vi "Tracer_ClassAttributes.vi"() -> ()   [LabVIEW 2018, in "TracerLibrary.lvlib" / "Tracer.lvclass"]
uses:
  Tracer.lvclass
  Tracer_ObjectAttributes.ctl
panel:
  in  "Max Input Size":i32=200
  in  "Enable Global Tracing":bool
  in  "UpdateCount":i32
  in  "Max Interal Trace Size":i32=-1
  in  "TraceQueues":refnum<queue>[](array[refnum])
  in  "Class Attributes":refnum<data-value>
  # "Trace items"
  # "VI start control trace"
  # "Queue data"
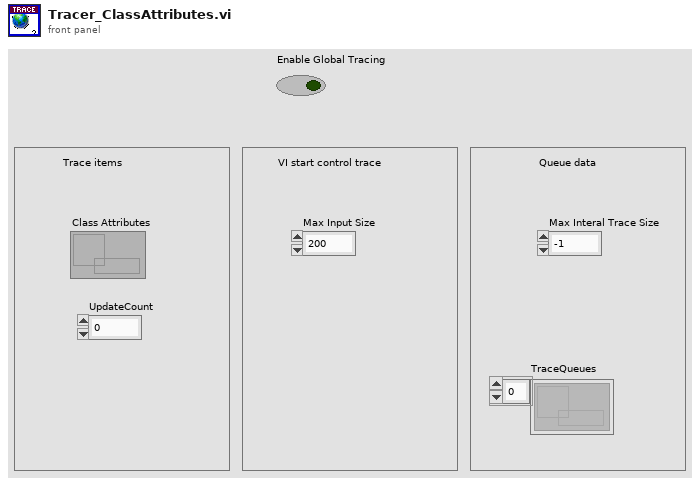
[diagram p1: front panel]
diagram:
